vi "fpga_FIFO control.vi"(0 "Time stamp":fxp<+,64,32> format="%.42g", 1 "reset":bool, 2 "nominal frequency":enum16{"50 Hz", "60 Hz"}(ring), 5 "Frequency":fxp<+,32,8>, 7 "#ch":fxp<+,5,5>, 9 "PMU VI input valid":bool, 11 "PMU VI output valid":bool) -> (4 "Time Stamp out":fxp<+,64,32> format="%.42g", 15 "Frequency output":fxp<+,32,8> format="%.27g")   [LabVIEW 2011, in "NI_EP_PMU_FPGA.lvlib"]
uses:
  <vilib>/addons/Electrical Power/PMU/NI_EP_PMU_FPGA.lvlib
  <vilib>/rvi/DataTransferAndStorage/Container/Common/niFpgaContainerState.ctl
  <vilib>/rvi/DataTransferAndStorage/Container/Common/niFpgaDataTypeControl.ctl
  <vilib>/rvi/DataTransferAndStorage/Container/Common/niFpgaContainerImplementationControl.ctl
  <vilib>/rvi/DataTransferAndStorage/Container/Common/niFpgaContainerArbitrationOptionsControl.ctl
  <vilib>/rvi/DataTransferAndStorage/Container/Common/niFpgaTransferTypeControl.ctl
  <vilib>/rvi/DataTransferAndStorage/Container/Common/niFpgaContainerInitializationParameters.ctl
  <vilib>/rvi/Memory/Memory_Types/niFpgaMemoryInterfaceConfiguration.ctl
  <vilib>/rvi/FIFO/Fifo_Types/niFpgaFifoControlLogicControl.ctl
  <vilib>/rvi/DataTransferAndStorage/Container/Common/niFpgaContainerMetaDataKey.ctl
  <vilib>/rvi/FXPMathLib/FxpSub/subVIs/nifxpmath_Sub_SimConfig.ctl
  <vilib>/fxp/LVFixedPointQuantizationPolicyTypeDef.ctl
  <vilib>/fxp/LVFixedPointOverflowPolicyTypeDef.ctl
  <vilib>/rvi/DataTransferAndStorage/Container/Common/niFpgaContainerGetUniqueNameForEmu.vi
  <vilib>/rvi/DataTransferAndStorage/Container/Common/niFpgaContainerSetEmuInfo.vi
  <vilib>/rvi/eio/common/nirviEmuReportErrorAndStop.vi
  <vilib>/rvi/FXPMathLib/FxpSub/simVIs/DllFxpSubTemp_sub.vi
  <vilib>/rvi/FIFO/Fifo_Resource/nirvififoEmulationSetSize.vi
  <vilib>/rvi/LocalResourceManager/LocalResourceManager.xnode
  <vilib>/rvi/FXPMathLib/FxpSub/XNode/nifxpmath_Sub.xnode
  <vilib>/rvi/DataTransferAndStorage/Container/XNode/niFpgaContainer.xnode
  <vilib>/rvi/FIFO/Fifo_Resource/nirvififoEmulationWrite.vi
  <vilib>/rvi/FXPMathLib/basic elements/FxpDiscreteDelay/XNode/nifxpmath_DiscreteDelay.xnode
  <vilib>/rvi/FIFO/Fifo_Resource/nirvififoEmulationRead.vi
  <vilib>/addons/Electrical Power/PQ/Resampling/NI_EP_Resample_FPGA.lvlib
types:
  T1 = cluster{"frequency":fxp<+,32,8>, "timestamp":fxp<+,64,32>}
  T2 = cluster{"frequency":fxp<+,32,8>, "timestamp":fxp<+,64,32>}[]
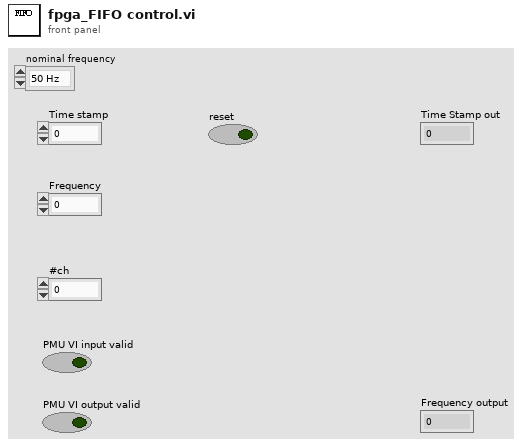
[diagram p1: front panel]
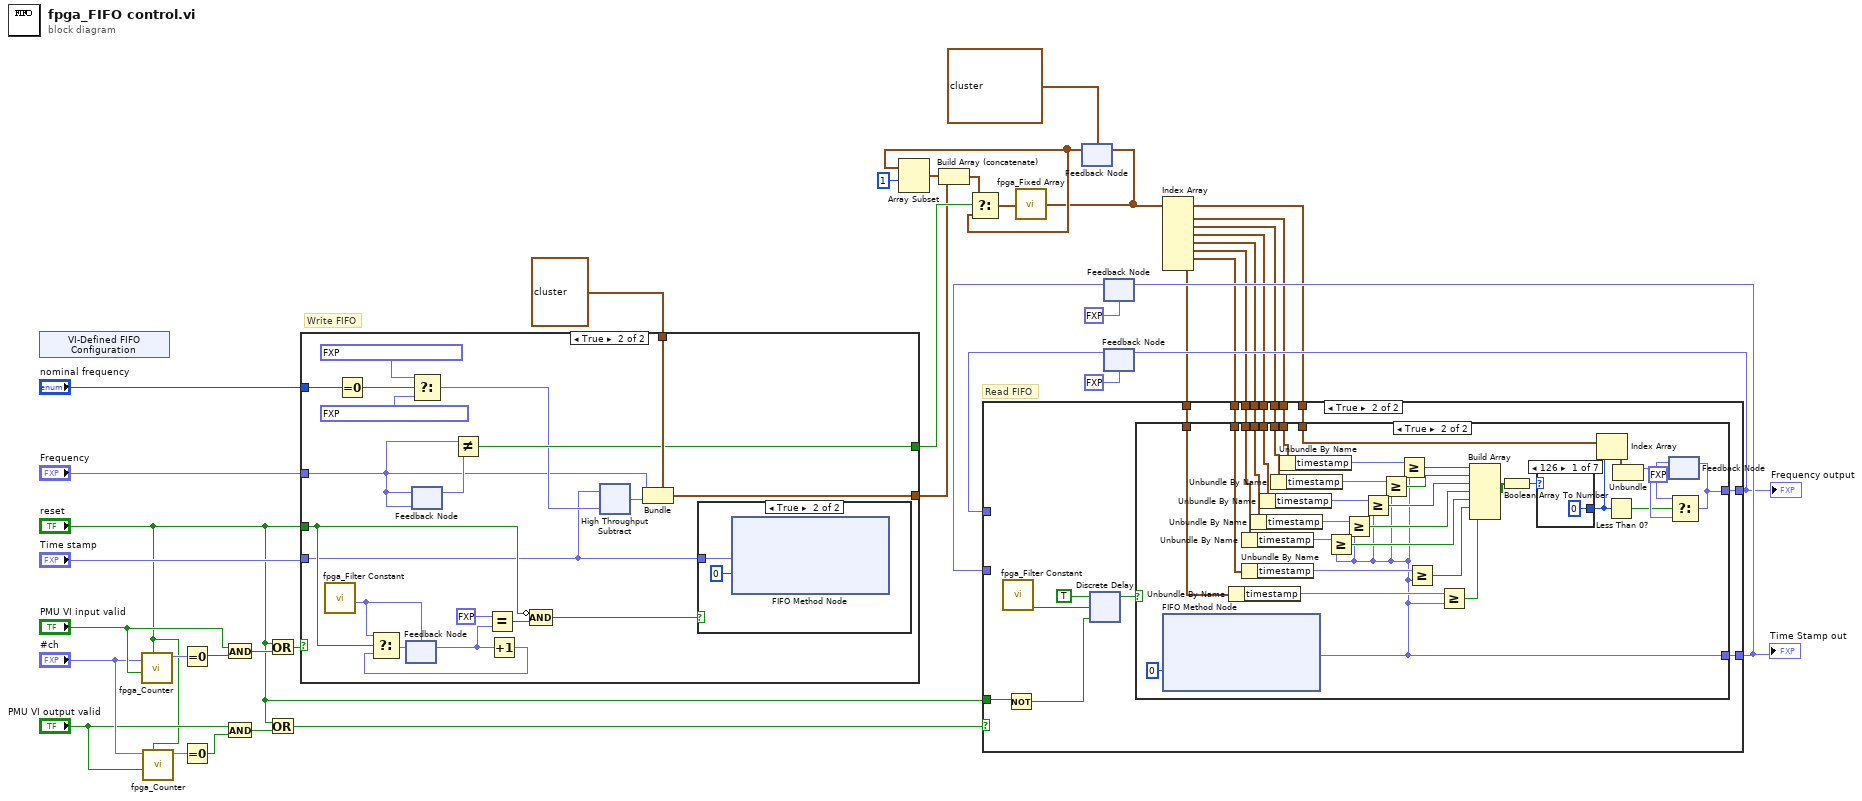
[diagram p0: block diagram]
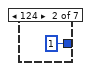
[diagram p4: hidden frame]
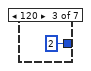
[diagram p5: hidden frame]
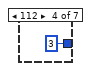
[diagram p6: hidden frame]
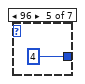
[diagram p7: hidden frame]
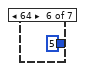
[diagram p8: hidden frame]
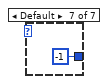
[diagram p9: hidden frame]
diagram:
  # "Read FIFO"
  # "Write FIFO"
  n1 = xnode "VI-Defined FIFO Configuration"() -> ()  [unwired: 1 out]
  n2 = call <vilib>:"fpga_Counter.vi"("reset"="reset", "Input Valid?"="PMU VI input valid", "upper limit"="#ch") -> ("count"=w25:fxp<+,5,5>)  [unwired: 7 in, 1 out]
  n3 = call <vilib>:"fpga_Counter.vi"("reset"="reset", "Input Valid?"="PMU VI output valid", "upper limit"="#ch") -> ("count"=w24:fxp<+,5,5>)  [unwired: 7 in, 1 out]
  n4 = Equal To 0?(x=w25) -> (x = 0?=w37:bool)
  n5 = Equal To 0?(x=w24) -> (x = 0?=w32:bool)
  n6 = And(x="PMU VI input valid", y=w37) -> (x .and. y?=w29:bool)
  n7 = And(x="PMU VI output valid", y=w32) -> (x .and. y?=w36:bool)
  n8 = Or(x="reset", y=w29) -> (x .or. y?=w28:bool)
  n9 = Or(x="reset", y=w36) -> (x .or. y?=w35:bool)
  n10 = case shown="True" w28 {
    tunnel: "Time stamp" -> [_ w40]
    tunnel: "reset" -> [_ w53]
    tunnel: "Frequency" -> [_ w39]
    tunnel: [_ w46] -> w16
    tunnel: [_ w48] -> w15
    tunnel: T1 {"frequency"=0.0, "timestamp"=0.0} -> [_ w47]
    tunnel: "nominal frequency" -> [_ w45]
    frame False {
    }
    frame True {
      n11 = call <vilib>:"fpga_Filter Constant.vi"() -> ("Start"=w52:fxp<+/-,4,4>)  [unwired: 8 in, 3 out]
      n12 = Equal To 0?(x=w45) -> (x = 0?=w44:bool)
      n13 = feedback #1(w52) -> (w56:fxp<+/-,4,4>)
      n14 = Select(t=fxp<+,18,-4> 0.060719966888427734 ("y"), s=w44, f=fxp<+,18,-4> 0.05672001838684082 ("y")) -> (s? t:f=w42:fxp<+,18,-4>)
      n15 = feedback #2(w39) -> (w50:fxp<+,32,8>)
      n16 = feedback-in #2(w39) -> ()
      n17 = Not Equal?(x=w39, y=w50) -> (x != y?=w46:bool)
      n18 = Equal?(x=fxp<+/-,4,4> 7.0, y=w56) -> (x = y?=w54:bool)
      n19 = Increment(x=w56) -> (x+1=w57:fxp<+,3,3>)
      n20 = Select(t=w52, s=w53, f=w57) -> (s? t:f=w58:fxp<+/-,4,4>)
      n21 = feedback-in #1(w58) -> ()
      n22 = Compound Arithmetic op=AND(invert w53, w54) -> (w51:bool)
      n23 = xnode "High Throughput Subtract"("x"=w40, "y"=w42) -> ("x-y"=w49:fxp<+,64,32>)
      n24 = Bundle(cluster=w47, "frequency"=w39, "timestamp"=w49) -> (w48:T1)
      n25 = case shown="True" w51 {
        tunnel: w40 -> [_ w86]
        frame False {
        }
        frame True {
          n26 = xnode ("FIFO Method Node")("Element"=w86, "Timeout"=0) -> ()  [unwired: 1 in, 2 out]
        }
      }
    }
  }
  n27 = feedback #3(T2 [{"frequency"=0.0, "timestamp"=0.0}, {"frequency"=0.0, "timestamp"=0.0}, {"frequency"=0.0, "timestamp"=0.0}, {"frequency"=0.0, "timestamp"=0.0}, {"frequency"=0.0, "timestamp"=0.0}, {"frequency"=0.0, "timestamp"=0.0}, {"frequency"=0.0, "timestamp"=0.0}]) -> (w3:T2)
  n28 = Array Subset(array=w3, index=1) -> (w17:T2)  [unwired: 1 in]
  n29 = Build Array (concatenate)(w17, w15) -> (w7:T2)
  n30 = Select(t=w7, s=w16, f=w3) -> (s? t:f=w6:T2)
  n31 = call <vilib>:"fpga_Fixed Array.vi"("Array"=w6) -> ("Array 2"=w2:T2)
  n32 = feedback-in #3(w2) -> ()
  n33 = feedback #4(fxp<+,64,32> 0.0 ("Element")) -> (w33:fxp<+,64,32>)
  n34 = feedback #5(fxp<+,32,8> 0.0 ("Element")) -> (w30:fxp<+,32,8>)
  n35 = Index Array(array=w2) -> (element #1=w14:T1, element #2=w13:T1, element #3=w12:T1, element #4=w11:T1, element #5=w10:T1, element #6=w5:T1, element #7=w4:T1)  [unwired: 7 in]
  n36 = case shown="True" w35 {
    tunnel: "reset" -> [_ w102]
    tunnel: [w89 w104] -> w34
    tunnel: w33 -> [w89 _]
    tunnel: [w88 w103] -> w20
    tunnel: w30 -> [w88 _]
    tunnel: w14 -> [_ w97]
    tunnel: w13 -> [_ w96]
    tunnel: w12 -> [_ w95]
    tunnel: w11 -> [_ w94]
    tunnel: w10 -> [_ w93]
    tunnel: w2 -> [_ w92]
    tunnel: w5 -> [_ w91]
    tunnel: w4 -> [_ w90]
    frame False {
    }
    frame True {
      n37 = call <vilib>:"fpga_Filter Constant.vi"() -> ("Total Delay"=w98:u8)  [unwired: 8 in, 3 out]
      n38 = Not(x=w102) -> (.not. x?=w100:bool)
      n39 = xnode "Discrete Delay"("D"=TRUE, "n-1[0..255]"=w98, "enable"=w100) -> ("Q"=w99:bool)
      n40 = case shown="True" w99 {
        tunnel: [_ w112] -> w104
        tunnel: [_ w107] -> w103
        tunnel: w97 -> [_ w132]
        tunnel: w96 -> [_ w133]
        tunnel: w95 -> [_ w134]
        tunnel: w94 -> [_ w135]
        tunnel: w93 -> [_ w136]
        tunnel: w92 -> [_ w126]
        tunnel: w91 -> [_ w117]
        tunnel: w90 -> [_ w114]
        frame False {
        }
        frame True {
          n41 = xnode ("FIFO Method Node")("Timeout"=0) -> ("Element"=w112:fxp<+,64,32>)  [unwired: 1 in, 2 out]
          n42 = Unbundle By Name(w114) -> ("timestamp"=w113:fxp<+,64,32>)
          n43 = Unbundle By Name(w136) -> ("timestamp"=w131:fxp<+,64,32>)
          n44 = Unbundle By Name(w117) -> ("timestamp"=w116:fxp<+,64,32>)
          n45 = Unbundle By Name(w135) -> ("timestamp"=w130:fxp<+,64,32>)
          n46 = Unbundle By Name(w134) -> ("timestamp"=w129:fxp<+,64,32>)
          n47 = Unbundle By Name(w133) -> ("timestamp"=w128:fxp<+,64,32>)
          n48 = Unbundle By Name(w132) -> ("timestamp"=w127:fxp<+,64,32>)
          n49 = Greater Or Equal?(x=w131, y=w112) -> (x >= y?=w121:bool)
          n50 = Greater Or Equal?(x=w130, y=w112) -> (x >= y?=w122:bool)
          n51 = Greater Or Equal?(x=w129, y=w112) -> (x >= y?=w123:bool)
          n52 = Greater Or Equal?(x=w128, y=w112) -> (x >= y?=w124:bool)
          n53 = Greater Or Equal?(x=w127, y=w112) -> (x >= y?=w125:bool)
          n54 = Greater Or Equal?(x=w116, y=w112) -> (x >= y?=w115:bool)
          n55 = Greater Or Equal?(x=w113, y=w112) -> (x >= y?=w111:bool)
          n56 = Build Array(w125, w124, w123, w122, w121, w115, w111) -> (w120:bool[])
          n57 = Boolean Array To Number(Boolean array=w120) -> (number=w119:u8)
          n58 = case shown="126" w119 {
            tunnel: [0 ("index") 1 ("index") 2 ("index") 3 ("index") 4 ("index") 5 ("index") -1 ("index")] -> w110
            frame 126 {
            }
            frame 124 {
            }
            frame 120 {
            }
            frame 112 {
            }
            frame 96 {
            }
            frame 64 {
            }
            frame Default {
            }
          }
          n59 = Index Array(array=w126, index=w110) -> (element=w118:T1)
          n60 = Less Than 0?(x=w110) -> (x < 0?=w106:bool)
          n61 = Unbundle(w118) -> ("frequency"=w109:fxp<+,32,8>)  [unwired: 1 out]
          n62 = feedback #6(fxp<+,32,8> 0.0 ("frequency")) -> (w108:fxp<+,32,8>)
          n63 = Select(t=w108, s=w106, f=w109) -> (s? t:f=w107:fxp<+,32,8>)
          n64 = feedback-in #6(w107) -> ()
        }
      }
    }
  }
  "Time Stamp out" <- w34
  "Frequency output" <- w20
  n65 = feedback-in #4(w34) -> ()
  n66 = feedback-in #5(w20) -> ()
